vi "My_AQ_AI.vi"() -> ()   [LabVIEW 2024]
uses:
  <vilib>/DAQmx/read.llb/DAQmx Read (Analog 1D Wfm NChan NSamp).vi
  <vilib>/DAQmx/create/channels.llb/DAQmx Create Channel (AI-Voltage-Basic).vi
  <vilib>/DAQmx/configure/timing.llb/DAQmx Timing (Sample Clock).vi
  <vilib>/DAQmx/miscellaneous.llb/DAQmx Fill In Error Info.vi
  <vilib>/Waveform/WDTOps.llb/WDT Index Channel DBL.vi
  <vilib>/Analysis/2dsp.llb/Decimate (continuous, DBL).vi
  <vilib>/Analysis/NI_AALPro.lvlib
panel:
  in  "factor decimacion":i32=20
  in  "tamaño buffer":i32=1000
  in  "Frecuencia muestreo":i32=20000
  in  "DAQmx Physical Channel":tag
  out "Senal EMG":waveform(dbl)[](graph)
  in  "Parar adquisicion":bool
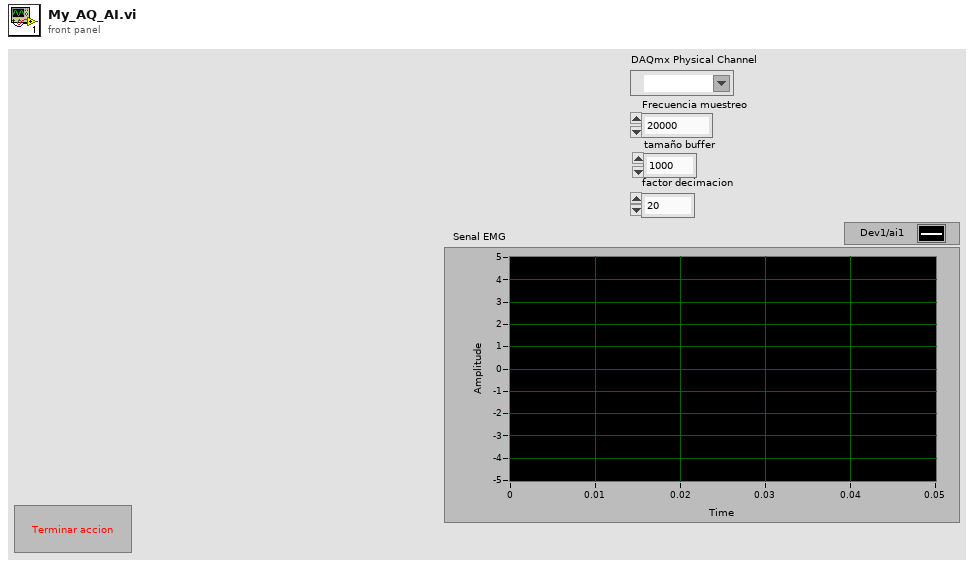
[diagram p1: front panel]
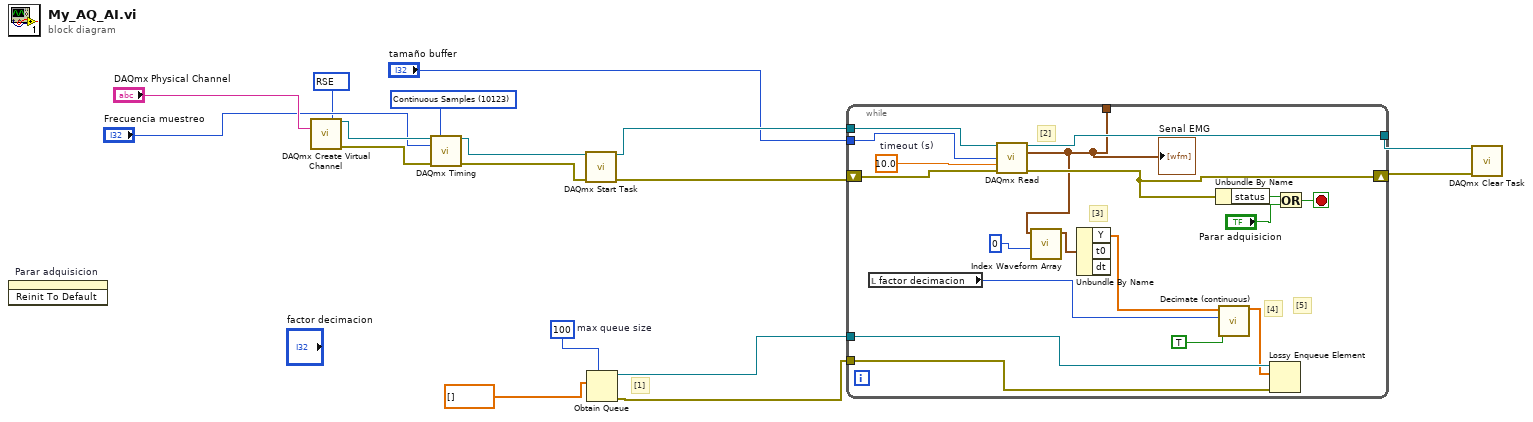
[diagram p0: block diagram]
diagram:
  w1 = 10123 items=["Finite Samples"=10178, "Continuous Samples"=10123, "Hardware Timed Single Point"=12522] ("sample mode")
  w2 = 10083 items=["Default"=-1, "RSE"=10083, "NRSE"=10078, "Differential"=10106, "Pseudodifferential"=12529] ("input terminal configuration")
  w12 = 100  # max queue size
  # "[1]"
  n1 = invoke on="Parar adquisicion" class="Bool (strict)" method="Reinit To Default"() -> ()  [unwired: 3 in, 3 out]
  n2 = call-poly <vilib>:"DAQmx Create Virtual Channel.vi"("input terminal configuration"=w2, "physical channels"="DAQmx Physical Channel") -> ("task out"=w8:refnum<k21>, "error out"=w7:errorcluster)  [unwired: 12 in]
  n3 = call-poly <vilib>:"DAQmx Timing.vi"("task/channels in"=w8, "sample mode"=w1, "rate"="Frecuencia muestreo", "error in"=w7) -> ("task out"=w6:refnum<k21>, "error out"=w5:errorcluster)  [unwired: 10 in]
  n4 = call <vilib>:"DAQmx Start Task.vi"("task/channels in"=w6, "error in"=w5) -> ("task out"=w17:refnum<k21>, "error out"=w16:errorcluster)  [unwired: 12 in]
  n5 = Obtain Queue(max queue size (-1, unlimited)=w12, element data type=dbl[] [] ("Cola tipo")) -> (queue out=w9:refnum<queue>, error out=w10:errorcluster)  [unwired: 3 in, 1 out]
  n6 = while {
    tunnel: w17 -> [w35]
    tunnel: "tamaño buffer" -> [w32]
    tunnel: [w33] -> w13
    shift-right: [w30] -> w14
    shift-left: w16 -> [w34]
    tunnel: [w24] -> _
    tunnel: w9 -> [w20]
    tunnel: w10 -> [w19]
    stop <- w29 stop-if-true
    w28 = 10.0  # timeout (s)
    # "[5]"
    # "[4]"
    # "[3]"
    # "[2]"
    n7 = local read "factor decimacion"() -> (w21:i32)
    n8 = call-poly <vilib>:"DAQmx Read.vi"("task/channels in"=w35, "number of samples per channel"=w32, "timeout"=w28, "error in"=w34) -> ("task out"=w33:refnum<k21>, "data"=w24:waveform(dbl)[], "error out"=w30:errorcluster)  [unwired: 9 in]
    "Senal EMG" <- w24
    n9 = call-poly <vilib>:"Index Waveform Array.vi"("index"=0, "waveform array"=w24) -> ("waveform"=w25:waveform(dbl))  [unwired: 8 in, 1 out]
    n10 = Unbundle By Name(w25) -> ("Y"=w22:dbl[])  [unwired: 2 out]
    n11 = Unbundle By Name(w30) -> ("status"=w31:bool)
    n12 = call-poly <vilib>:"Decimate (continuous).vi"("averaging"=TRUE, "decimating factor"=w21, "X"=w22) -> ("Decimated Array"=w18:dbl[])  [unwired: 7 in, 1 out]
    n13 = Lossy Enqueue Element(queue=w20, element=w18, error in (no error)=w19) -> ()  [unwired: 4 out]
    n14 = Or(x=w31, y="Parar adquisicion") -> (x .or. y?=w29:bool)
  }
  n15 = call <vilib>:"DAQmx Clear Task.vi"("task in"=w13, "error in"=w14) -> ()  [unwired: 13 in, 1 out]
